vi "JKISM++ Call and Monitor TCP Traffic.vi"() -> ()   [LabVIEW 2014]
uses:
  user.lib/_NEVSTOP/JKI State Machine++/JKI State Machine++.lvlib
panel:
  in  "String":string
  out "String Cache":string
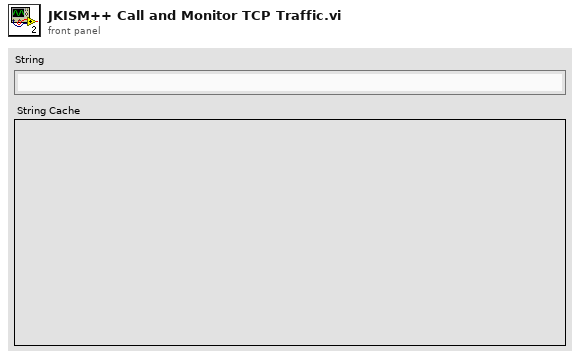
[diagram p1: front panel]
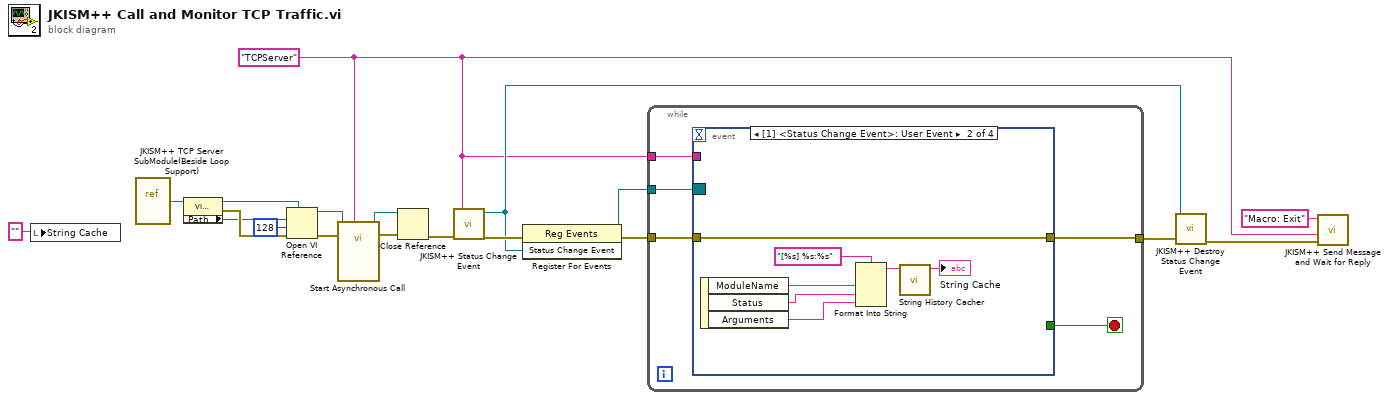
[diagram p0: block diagram]
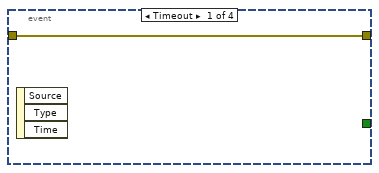
[diagram p2: hidden frame]
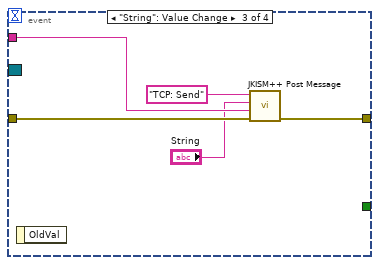
[diagram p3: hidden frame]
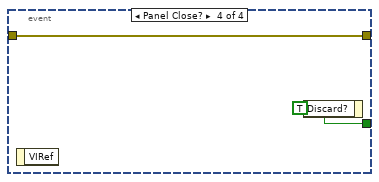
[diagram p4: hidden frame]
diagram:
  w3 = "TCPServer" ("Name(\"\" to use uuid)")
  n1 = local write "String Cache"("" ("String Cache")) -> ()
  n2 = vi-ref "JKISM++ TCP Server SubModule(Beside Loop Support).vi"() -> (w12:refnum<vi>)
  n3 = property class="VI (strict)"(reference=w12) -> (reference out=w16:refnum<vi>, error out=w14:errorcluster, "Path"=w13:path)  [unwired: 1 in]
  n4 = Open VI Reference(type specifier VI Refnum (for type only)=w16, vi path=w13, options=128, error in (no error)=w14) -> (vi reference=w15:refnum<vi>, error out=w11:errorcluster)  [unwired: 2 in]
  n5 = call-by-ref "Start Asynchronous Call"(reference=w15, error in=w11, "Name(\"\" to use uuid)"=w3) -> (reference out=w18:refnum<vi>, error out=w17:errorcluster)  [unwired: 11 in]
  n6 = Close Reference(reference=w18, error in (no error)=w17) -> (error out=w10:errorcluster)
  n7 = call "JKISM++ Status Change Event.vi"("Error in"=w10, "Name(\"\" to use uuid) in"=w3) -> ("Error out"=w9:errorcluster, "Status Change Event"=w5:refnum<user-event>)  [unwired: 8 in]
  n8 = register-events(error in=w9, w5) -> (reference out=w7:refnum<event-registration>, error out=w8:errorcluster)  [unwired: 1 in]
  n9 = while {
    tunnel: w8 -> [w21]
    tunnel: w7 -> [w23]
    tunnel: [w22] -> w6
    tunnel: w3 -> [w20]
    stop <- w24 stop-if-true
    n10 = event shown="[1] <Status Change Event>: User Event" {
      selector: w23 -> [_ _ _ _]
      dyn-events: _ -> [_ _ _ _]
      timeout: _ -> [_ _ _ _]
      tunnel: [_ _ _ w39] -> w24
      tunnel: [w25 w32 w36 w38] -> w22
      tunnel: w21 -> [w25 w32 w37 w38]
      tunnel: w20 -> [_ _ w35 _]
      event Timeout {
        n11 = event-data() -> ()  [unwired: 1 in, 3 out]
      }
      event User Event {
        n12 = event-data() -> ("ModuleName"=w31:string, "Status"=w30:string, "Arguments"=w29:string)  [unwired: 1 in]
        n13 = Format Into String(format string="[%s] %s:%s", w31, w30, w29) -> (resulting string=w27:string)  [unwired: 2 in, 1 out]
        n14 = call "String History Cacher.vi"("String"=w27) -> ("String Cache"=→"String Cache":string)  [unwired: 10 in]
      }
      event "String": Value Change {
        n15 = event-data() -> ()  [unwired: 1 in, 1 out]
        n16 = call "JKISM++ Post Message.vi"("Error In (no error)"=w37, "Target Module"=w35, "Arguments (\"\")"="String", "State"="TCP: Send") -> ("error out"=w36:errorcluster)  [unwired: 7 in]
      }
      event Panel Close? {
        w39 = TRUE ("Discard?")
        n17 = event-data() -> ()  [unwired: 1 in, 1 out]
        n18 = event-data("Discard?"=w39) -> ()  [unwired: 1 in, 1 out]
      }
    }
  }
  n19 = call "JKISM++ Destroy Status Change Event.vi"("Error in"=w6, "Status Change Event"=w5) -> ("Error out"=w4:errorcluster)  [unwired: 9 in]
  n20 = call "JKISM++ Send Message and Wait for Reply.vi"("Error In (no error)"=w4, "Target Module"=w3, "State"="Macro: Exit") -> ()  [unwired: 7 in, 2 out]
